vi "fpga_Previous Timestamp.vi"(8 "input valid? (T)":bool=TRUE, 10 "channel index":u8, 11 "timestamp":u32) -> (3 "previous timestamp":u32)   [LabVIEW 2012, in "NI_EP_Protection_FPGA.lvlib"]
uses:
  <vilib>/addons/Electrical Power/Protection/NI_EP_Protection_FPGA.lvlib
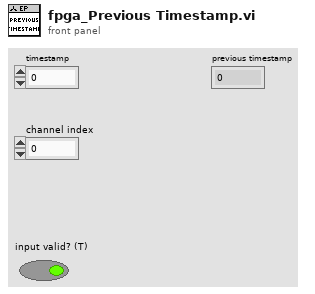
[diagram p1: front panel]
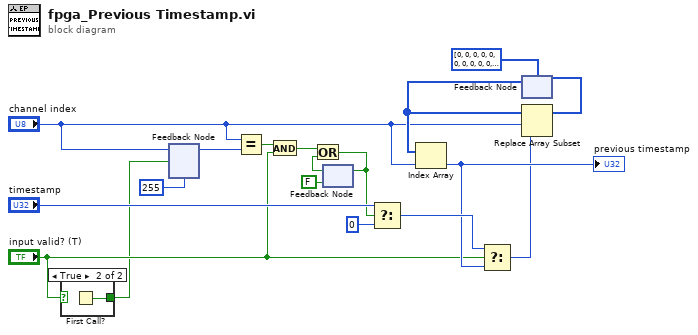
[diagram p0: block diagram]
diagram:
  n1 = case shown="True" "input valid? (T)" {
    tunnel: [_ w19] -> w1
    frame False {
    }
    frame True {
      n2 = First Call?() -> (First Call?: T/F=w19:bool)
    }
  }
  n3 = feedback #1(u8 255 ("channel index")) -> (w15:u8)
  n4 = feedback-in #1("channel index", w1) -> ()
  n5 = Equal?(x="channel index", y=w15) -> (x = y?=w11:bool)
  n6 = And(x=w11, y="input valid? (T)") -> (x .and. y?=w10:bool)
  n7 = feedback #2(FALSE) -> (w9:bool)
  n8 = Or(x=w10, y=w9) -> (x .or. y?=w7:bool)
  n9 = feedback-in #2(w7) -> ()
  n10 = Select(t="timestamp", s=w7, f=u32 0 ("timestamp [s]")) -> (s? t:f=w6:u32)
  n11 = feedback #3(u32[] [0, 0, 0, 0, 0, 0, 0, 0, 0, 0, 0, 0, 0, 0, 0, 0]) -> (w18:u32[])
  n12 = Index Array(array=w18, index="channel index") -> (element=w5:u32)
  "previous timestamp" <- w5
  n13 = Select(t=w6, s="input valid? (T)", f=w5) -> (s? t:f=w4:u32)
  n14 = Replace Array Subset(array=w18, new element=w4, index="channel index") -> (w3:u32[])
  n15 = feedback-in #3(w3) -> ()
